vi "UserVars-Draw From Random Distribution.vi"(0 "Expr in":string, 7 "Nrand":i32=1, 11 "error in (no error)":errorcluster) -> (4 "Expr out":string, 15 "error out":errorcluster)   [LabVIEW 2020]
uses:
  <vilib>/gmath/statdist.llb/Normal Random.vi
  <vilib>/gmath/statdist.llb/Exp Random.vi
  <vilib>/gmath/statdist.llb/Uniform Random.vi
  <vilib>/regexp/Match Regular Expression.xnode
  <vilib>/gmath/NI_Gmath.lvlib
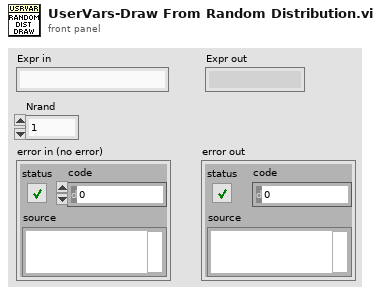
[diagram p1: front panel]
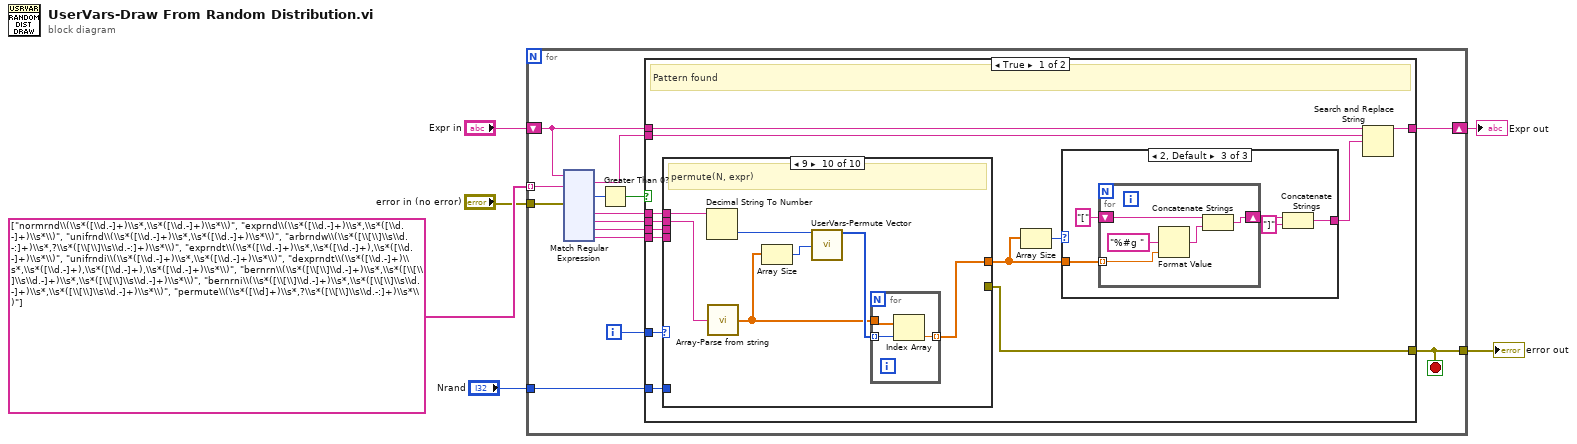
[diagram p0: block diagram]
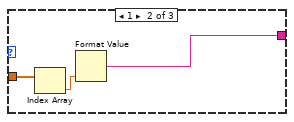
[diagram p3: hidden frame]
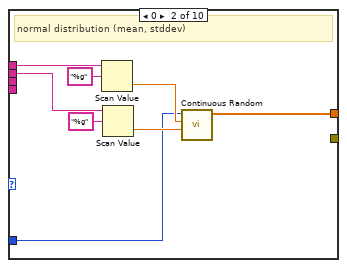
[diagram p5: hidden frame]
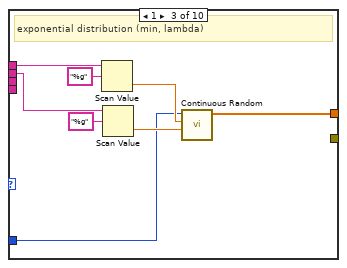
[diagram p6: hidden frame]
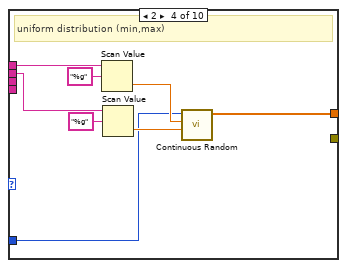
[diagram p7: hidden frame]
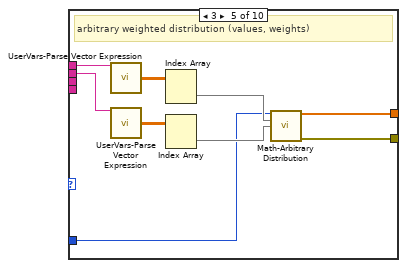
[diagram p8: hidden frame]
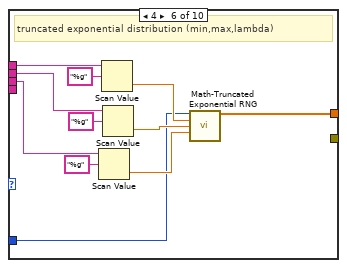
[diagram p9: hidden frame]
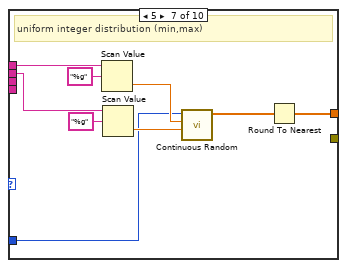
[diagram p10: hidden frame]
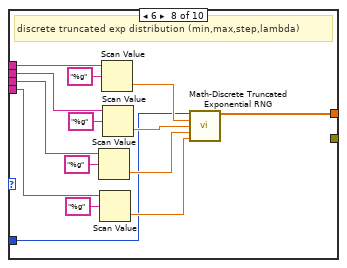
[diagram p11: hidden frame]
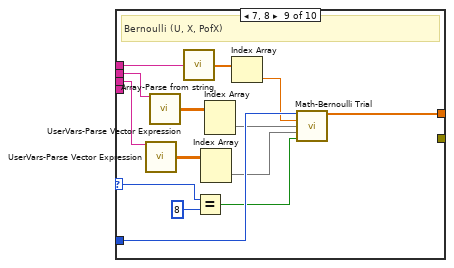
[diagram p12: hidden frame]
diagram:
  n1 = for {
    shift-right: [w17] -> w3
    shift-left: "Expr in" -> [w18]
    tunnel: string[] ["normrnd\\(\\s*([\\d.-]+)\\s*,\\s*([\\d.-]+)\\s*\\)", "exprnd\\(\\s*([\\d.-]+)\\s*,\\s*([\\d.-]+)\\s*\\)", "unifrnd\\(\\s*([\\d.-]+)\\s*,\\s*([\\d.-]+)\\s*\\)", "arbrndw\\(\\s*([\\[\\]\\s\\d.-:]+)\\s*,?\\s*([\\[\\]\\s\\d.-:]+)\\s*\\)", "exprndt\\(\\s*([\\d.-]+)\\s*,\\s*([\\d.-]+),\\s*([\\d.-]+)\\s*\\)", "unifrndi\\(\\s*([\\d.-]+)\\s*,\\s*([\\d.-]+)\\s*\\)", "dexprndt\\(\\s*([\\d.-]+)\\s*,\\s*([\\d.-]+),\\s*([\\d.-]+),\\s*([\\d.-]+)\\s*\\)", "bernrn\\(\\s*([\\[\\]\\d.-]+)\\s*,\\s*([\\[\\]\\s\\d.-]+)\\s*,\\s*([\\[\\]\\s\\d.-]+)\\s*\\)", "bernrni\\(\\s*([\\[\\]\\d.-]+)\\s*,\\s*([\\[\\]\\s\\d.-]+)\\s*,\\s*([\\[\\]\\s\\d.-]+)\\s*\\)", "permute\\(\\s*([\\d]+)\\s*,?\\s*([\\[\\]\\s\\d.-:]+)\\s*\\)"] ("String") -> [w9] mode=indexing
    tunnel: "error in (no error)" -> [w20]
    tunnel: [w10] -> w2
    tunnel: "Nrand" -> [w7]
    i -> [w12]
    stop <- w10 stop-if-true
    n2 = xnode "Match Regular Expression"("input string"=w18, "regular expression"=w9, "error in"=w20) -> ("whole match"=w16:string, "offset past match"=w19:i32, "submatch 1"=w15:string, "submatch 2"=w14:string, "submatch 3"=w11:string, "submatch 4"=w8:string)  [unwired: 3 in, 3 out]
    n3 = Greater Than 0?(x=w19) -> (x > 0?=w13:bool)
    n4 = case shown="True" w13 {
      tunnel: w18 -> [w28 w138]
      tunnel: [w25 w138] -> w17
      tunnel: w16 -> [w27 _]
      tunnel: w15 -> [w32 _]
      tunnel: w14 -> [w31 _]
      tunnel: w12 -> [w33 _]
      tunnel: w11 -> [w30 _]
      tunnel: [w29 _] -> w10
      tunnel: w8 -> [w24 _]
      tunnel: w7 -> [w23 _]
      frame True {
        # "Pattern found"
        n5 = case shown="9" w33 {
          selector: w33 -> [_ _ _ _ _ _ _ _ w119 _]
          tunnel: w32 -> [_ w54 w62 w70 w79 w90 w99 w113 w116 w133]
          tunnel: w31 -> [_ w51 w59 w67 w76 w87 w96 w110 w124 w134]
          tunnel: [_ w48 w56 w66 w73 w81 w93 w105 w127 w130] -> w21
          tunnel: w30 -> [_ _ _ _ _ w85 _ w108 w121 _]
          tunnel: [_ _ _ _ w72 _ _ _ _ _] -> w29
          tunnel: w24 -> [_ _ _ _ _ _ _ w103 _ _]
          tunnel: w23 -> [_ w47 w55 w63 w71 w80 w92 w100 w126 _]
          frame -1, Default {
          }
          frame 0 {
            # "normal distribution (mean, stddev)"
            n6 = Scan Value(string=w54, format string="%g") -> (value=w50:dbl)  [unwired: 1 in, 1 out]
            n7 = Scan Value(string=w51, format string="%g") -> (value=w49:dbl)  [unwired: 1 in, 1 out]
            n8 = call-poly <vilib>:"Continuous Random.vi"("std"=w49, "mean"=w50, "samples"=w47) -> ("normal random data"=w48:dbl[])  [unwired: 7 in, 1 out]
          }
          frame 1 {
            # "exponential distribution (min, lambda)"
            n9 = Scan Value(string=w62, format string="%g") -> (value=w58:dbl)  [unwired: 1 in, 1 out]
            n10 = Scan Value(string=w59, format string="%g") -> (value=w57:dbl)  [unwired: 1 in, 1 out]
            n11 = call-poly <vilib>:"Continuous Random.vi"("b"=w57, "a"=w58, "samples"=w55) -> ("exp random data"=w56:dbl[])  [unwired: 7 in, 1 out]
          }
          frame 2 {
            # "uniform distribution (min,max)"
            n12 = Scan Value(string=w70, format string="%g") -> (value=w65:dbl)  [unwired: 1 in, 1 out]
            n13 = Scan Value(string=w67, format string="%g") -> (value=w64:dbl)  [unwired: 1 in, 1 out]
            n14 = call-poly <vilib>:"Continuous Random.vi"("xmax"=w64, "xmin"=w65, "samples"=w63) -> ("uniform random data"=w66:dbl[])  [unwired: 7 in, 1 out]
          }
          frame 3 {
            # "arbitrary weighted distribution (values, weights)"
            n15 = call "UserVars-Parse Vector Expression.vi"("Expression In"=w79) -> ("values"=w78:dbl[][])  [unwired: 11 in, 3 out]
            n16 = call "UserVars-Parse Vector Expression.vi"("Expression In"=w76) -> ("values"=w77:dbl[][])  [unwired: 11 in, 3 out]
            n17 = Index Array(array=w78) -> (element=w75:dbl[])  [unwired: 2 in]
            n18 = Index Array(array=w77) -> (element=w74:dbl[])  [unwired: 2 in]
            n19 = call "Math-Arbitrary Distribution.vi"("samples"=w71, "Values"=w75, "Weights"=w74) -> ("Array"=w73:dbl[], "error out"=w72:errorcluster)  [unwired: 11 in]
          }
          frame 4 {
            # "truncated exponential distribution (min,max,lambda)"
            n20 = Scan Value(string=w85, format string="%g") -> (value=w82:dbl)  [unwired: 1 in, 1 out]
            n21 = Scan Value(string=w90, format string="%g") -> (value=w84:dbl)  [unwired: 1 in, 1 out]
            n22 = Scan Value(string=w87, format string="%g") -> (value=w83:dbl)  [unwired: 1 in, 1 out]
            n23 = call "Math-Truncated Exponential RNG.vi"("samples"=w80, "Min"=w84, "Max"=w83, "Lambda"=w82) -> ("Array"=w81:dbl[])  [unwired: 11 in]
          }
          frame 5 {
            # "uniform integer distribution (min,max)"
            n24 = Scan Value(string=w99, format string="%g") -> (value=w95:dbl)  [unwired: 1 in, 1 out]
            n25 = Scan Value(string=w96, format string="%g") -> (value=w94:dbl)  [unwired: 1 in, 1 out]
            n26 = call-poly <vilib>:"Continuous Random.vi"("xmax"=w94, "xmin"=w95, "samples"=w92) -> ("uniform random data"=w91:dbl[])  [unwired: 7 in, 1 out]
            n27 = Round To Nearest(number=w91) -> (nearest integer value=w93:dbl[])
          }
          frame 6 {
            # "discrete truncated exp distribution (min,max,step,lambda)"
            n28 = Scan Value(string=w108, format string="%g") -> (value=w102:dbl)  [unwired: 1 in, 1 out]
            n29 = Scan Value(string=w103, format string="%g") -> (value=w101:dbl)  [unwired: 1 in, 1 out]
            n30 = Scan Value(string=w113, format string="%g") -> (value=w107:dbl)  [unwired: 1 in, 1 out]
            n31 = Scan Value(string=w110, format string="%g") -> (value=w106:dbl)  [unwired: 1 in, 1 out]
            n32 = call "Math-Discrete Truncated Exponential RNG.vi"("samples"=w100, "Min"=w107, "Max"=w106, "Step"=w102, "Lambda"=w101) -> ("Array"=w105:dbl[])  [unwired: 10 in]
          }
          frame 7, 8 {
            # "Bernoulli (U, X, PofX)"
            n33 = call "UserVars-Parse Vector Expression.vi"("Expression In"=w121) -> ("values"=w122:dbl[][])  [unwired: 11 in, 3 out]
            n34 = call "UserVars-Parse Vector Expression.vi"("Expression In"=w124) -> ("values"=w125:dbl[][])  [unwired: 11 in, 3 out]
            n35 = call "Array-Parse from string.vi"("String"=w116) -> ("Array"=w115:dbl[])  [unwired: 13 in, 1 out]
            n36 = Equal?(x=w119, y=8) -> (x = y?=w117:bool)
            n37 = Index Array(array=w122) -> (element=w120:dbl[])  [unwired: 2 in]
            n38 = Index Array(array=w125) -> (element=w123:dbl[])  [unwired: 2 in]
            n39 = Index Array(array=w115) -> (element=w114:dbl)  [unwired: 1 in]
            n40 = call "Math-Bernoulli Trial.vi"("samples"=w126, "U"=w114, "X"=w123, "PofX"=w120, "interpolate"=w117) -> ("Array"=w127:dbl[])  [unwired: 9 in, 1 out]
          }
          frame 9 {
            # "permute(N, expr)"
            n41 = Decimal String To Number(string=w133) -> (number=w132:i32)  [unwired: 2 in, 1 out]
            n42 = call "Array-Parse from string.vi"("String"=w134) -> ("Array"=w129:dbl[])  [unwired: 13 in, 1 out]
            n43 = Array Size(array=w129) -> (size(s)=w128:i32)
            n44 = call "UserVars-Permute Vector.vi"("Seed"=w132, "N"=w128) -> ("Array"=w131:i32[])  [unwired: 12 in, 1 out]
            n45 = for {
              tunnel: w129 -> [w137]
              tunnel: w131 -> [w136] mode=indexing
              tunnel: [w135] -> w130 mode=indexing
              n46 = Index Array(array=w137, index=w136) -> (element=w135:dbl)
            }
          }
        }
        n47 = Array Size(array=w21) -> (size(s)=w22:i32)
        n48 = case shown="2, Default" w22 {
          tunnel: [_ w36 w37] -> w26
          tunnel: w21 -> [_ w35 w41]
          frame 0 {
          }
          frame 1 {
            n49 = Index Array(array=w35) -> (element=w34:dbl)  [unwired: 1 in]
            n50 = Format Value(value (0)=w34) -> (output string=w36:string)  [unwired: 2 in]
          }
          frame 2, Default {
            n51 = for {
              tunnel: w41 -> [w46] mode=indexing
              shift-right: [w44] -> w39
              shift-left: "[" -> [w43]
              n52 = Format Value(format string="%#g ", value (0)=w46) -> (output string=w42:string)  [unwired: 1 in]
              n53 = Concatenate Strings(w43, w42) -> (w44:string)
            }
            n54 = Concatenate Strings(w39, "]" ("string")) -> (w37:string)
          }
        }
        n55 = Search and Replace String(input string=w28, search string=w27, replace string=w26) -> (result string=w25:string)  [unwired: 5 in, 3 out]
      }
      frame False {
      }
    }
  }
  "error out" <- w2
  "Expr out" <- w3
